vi "UHR-Fleezers Control (host) - Lorentz v2.vi"() -> ()   [LabVIEW 2014] (continued)
          shift-right: [w1383] -> _
          shift-left: 0.0 -> [w1381]
          i -> [w1390]
          stop <- w1454 stop-if-true
          w1398 = 0 ("index")
          w1419 = 1 ("dimension size")
          # "Keep phase within\n2pi so errors don't \nbuild"
          # "Accumulated\nphase"
          # "Current phase"
          # "Trap 2"
          # "Trap 1"
          # "ignore if N = 0"
          # "r"
          # "r"
          # "r"
          # "r"
          # "\"omega*t\""
          # "Trap 2"
          # "Trap separation (radians)"
          # "Trap 1"
          # "Offset (starts\n at bottom of\n the circle)"
          # "omega"
          n833 = node-c288() -> (w1467:i64)  [unwired: 1 in]
          n834 = Divide(x=w1467, y=1000) -> (x/y=w1386:dbl)
          n835 = Divide(x="2D Motion Trap Separation (MHz)", y="Radius (MHz)") -> (x/y=w1441:dbl)
          n836 = Negate(x=w1386) -> (-x=w1385:dbl)
          n837 = Divide(x="Trap 2 phase shift (deg)", y=360.0) -> (x/y=w1432:dbl)
          n838 = Inverse Sine(1:w1441) -> (0:w1377:dbl)
          n839 = Multiply(x=6.283185307179586, y=w1432) -> (x*y=w1378:dbl)
          n840 = Multiply(x=6.283185307179586, y="2D Motion Frequency (Hz)") -> (x*y=w1389:dbl)
          n841 = Select(t=w1386, s="Counterclockwise/Clockwise", f=w1385) -> (s? t:f=w1388:dbl)
          n842 = Multiply(x=w1389, y=w1388) -> (x*y=w1379:dbl)
          n843 = Select(t=w1377, s="Trap shift\nmethod", f=w1378) -> (s? t:f=w1376:dbl)
          n844 = Add(x=w1379, y=w1381) -> (x+y=w1382:dbl)
          n845 = Add(x=w1382, y=w1376) -> (x+y=w1438:dbl)
          n846 = Add(x=w1382, y=1.5707963267948966) -> (x+y=w1387:dbl)
          n847 = Add(x=w1438, y=1.5707963267948966) -> (x+y=w1451:dbl)
          n848 = Cosine(x=w1387) -> (cos(x)=w1465:dbl)
          n849 = Sine(x=w1387) -> (sin(x)=w1464:dbl)
          n850 = Multiply(x=w1465, y="Radius (MHz)") -> (x*y=w1458:dbl)
          n851 = Cosine(x=w1451) -> (cos(x)=w1463:dbl)
          n852 = Sine(x=w1451) -> (sin(x)=w1462:dbl)
          n853 = Multiply(x=w1464, y="Radius (MHz)") -> (x*y=w1457:dbl)
          n854 = Multiply(x=w1463, y="Radius (MHz)") -> (x*y=w1461:dbl)
          n855 = Multiply(x=w1462, y="Radius (MHz)") -> (x*y=w1459:dbl)
          n856 = Add(x=w1458, y=w1456) -> (x+y=w1407:dbl)
          n857 = Add(x=w1457, y=w1449) -> (x+y=w1405:dbl)
          n858 = Greater Or Equal?(x=w1390, y="N steps then stop") -> (x >= y?=w1448:bool)
          n859 = Add(x=w1461, y=w1460) -> (x+y=w1396:dbl)
          n860 = Add(x=w1459, y=w1449) -> (x+y=w1394:dbl)
          n861 = Not Equal To 0?(x="N steps then stop") -> (x != 0?=w1444:bool)
          n862 = And(x=w1448, y=w1444) -> (x .and. y?=w1445:bool)
          n863 = local read "Trap 1 sum mean"() -> (w1428:dbl)
          n864 = local read "Stop All"() -> (w1453:bool)
          n865 = local write "BD 1 Frequency 1 (MHz)"(w1407) -> ()
          n866 = local write "BD 2 Frequency 1 (MHz)"(w1405) -> ()
          n867 = local write "BD 1 Frequency 2 (MHz)"(w1396) -> ()
          n868 = local write "BD 2 Frequency 2 (MHz)"(w1394) -> ()
          n869 = Select(t=w1390, s="test", f=w1428) -> (s? t:f=→"Waveform Chart":dbl)
          n870 = Compound Arithmetic op=OR(w1453, "Stop Moving", w1445) -> (w1454:bool)
          n871 = local read "BD 1 Frequency 3 (MHz)"() -> (w1437:dbl)
          n872 = local read "BD 2 Frequency 3 (MHz)"() -> (w1436:dbl)
          n873 = Select(t=w1412, s="Reset graph", f=w1413) -> (s? t:f=w1393:dbl[])
          n874 = Select(t=w1412, s="Reset graph", f=w1414) -> (s? t:f=w1395:dbl[])
          n875 = Select(t=w1412, s="Reset graph", f=w1416) -> (s? t:f=w1404:dbl[])
          n876 = Select(t=w1412, s="Reset graph", f=w1417) -> (s? t:f=w1406:dbl[])
          n877 = Initialize Array(w1394, w1419) -> (w1420:dbl[])
          n878 = Initialize Array(w1405, w1419) -> (w1423:dbl[])
          n879 = Initialize Array(w1396, w1419) -> (w1421:dbl[])
          n880 = Initialize Array(w1407, w1419) -> (w1424:dbl[])
          n881 = local read "Y RF Frequency Limits (MHz)"() -> (w1434:T20)
          n882 = local read "X RF Frequency Limits (MHz)"() -> (w1435:T20)
          n883 = call "set RF board frequency - interlace.vi"("Board 2 Frequency Limits"=w1434, "Board 1 Frequency Limits"=w1435, "FPGA VI Reference In"=w1431, "Board 2 Frequency 3 (MHz)"=w1436, "Board 1 Frequency 3 (MHz)"=w1437, "Board 2 Frequency 2 (MHz)"=w1394, "Board 2 Frequency 1 (MHz)"=w1405, "Board 1 Frequency 2 (MHz)"=w1396, "Board 1 Frequency 1  (MHz)"=w1407) -> ()  [unwired: 1 in, 2 out]
          n884 = Bundle(w1421, w1420) -> (w1392:cluster{dbl[], dbl[]})  [unwired: 1 in]
          n885 = Bundle(w1424, w1423) -> (w1422:cluster{dbl[], dbl[]})  [unwired: 1 in]
          n886 = Build Array (concatenate)(w1407, w1406) -> (w1411:dbl[])
          n887 = Build Array (concatenate)(w1405, w1404) -> (w1409:dbl[])
          n888 = Build Array (concatenate)(w1396, w1395) -> (w1402:dbl[])
          n889 = Build Array (concatenate)(w1394, w1393) -> (w1400:dbl[])
          n890 = Bundle(w1411, w1409) -> (w1391:cluster{dbl[], dbl[]})  [unwired: 1 in]
          n891 = Bundle(w1402, w1400) -> (w1418:cluster{dbl[], dbl[]})  [unwired: 1 in]
          n892 = Build Array(w1422, w1392, w1391, w1418) -> (→"Trap trajectories":cluster{dbl[], dbl[]}[])
          n893 = case "To pause the process" shown="True" "Pause rotation" {
            frame False {
            }
            frame True {
              n894 = while {
                stop <- w1470 stop-if-true
                n895 = local read "Pause rotation"() -> (w1471:bool)
                n896 = Wait (ms)(milliseconds to wait=u32 10) -> ()  [unwired: 1 out]
                n897 = Not(x=w1471) -> (.not. x?=w1470:bool)
              }
            }
          }
          n898 = Decrement(x="N steps to plot") -> (x-1=w1397:i32)
          n899 = Array Subset(array=w1409, index=w1398, length=w1397) -> (w1408:dbl[])
          n900 = Array Subset(array=w1411, index=w1398, length=w1397) -> (w1410:dbl[])
          n901 = Array Subset(array=w1402, index=w1398, length=w1397) -> (w1401:dbl[])
          n902 = Array Subset(array=w1400, index=w1398, length=w1397) -> (w1399:dbl[])
          n903 = Quotient & Remainder(x=w1382, y=6.283185307179586) -> (x-y*floor(x/y)=w1383:dbl)  [unwired: 1 out]
          n904 = node-c288() -> ()  [unwired: 1 in, 1 out]
        }
        n905 = node-c288(w1363) -> ()  [unwired: 1 out]
        n906 = case shown="True" w1354 {
          tunnel: w1358 -> [_ w1369]
          tunnel: w1357 -> [_ w1368]
          tunnel: w1356 -> [_ w1367]
          tunnel: w1355 -> [_ w1366]
          frame False {
          }
          frame True {
            n907 = flat-sequence {
              tunnel: w1369 -> [w1373]
              tunnel: w1368 -> [w1372]
              tunnel: w1367 -> [w1371]
              tunnel: w1366 -> [w1370]
              frame #0 {
                n908 = local write "BD 1 Frequency 1 (MHz)"(w1373) -> ()
                n909 = local write "BD 2 Frequency 1 (MHz)"(w1372) -> ()
                n910 = local write "BD 1 Frequency 2 (MHz)"(w1371) -> ()
                n911 = local write "BD 2 Frequency 2 (MHz)"(w1370) -> ()
              }
              frame #1 {
                n912 = property on="Update all trap values" class="Bool (strict)"("Val(Sgnl)"=TRUE ("Value (Signaling)")) -> ()  [unwired: 2 in, 2 out]
              }
            }
          }
        }
      }
      event "Stop All": Value Change {
        # "Stopping blue laser before shutting off program"
        n913 = event-data() -> ()  [unwired: 1 in, 5 out]
        n914 = local read "Delay (ms)"() -> (w1481:i32)
        n915 = call "serial write macro.vi"("String"="l0", "Delay (ms)"=w1481, "VISA resource name"=w1484) -> ("read buffer"=w1479:string, "error out"=w1480:errorcluster, "VISA resource name out"=w1483:refnum<visa-resource-name>)
        n916 = local write "read blue buffer"(w1479) -> ()
        n917 = local write "Blue Error Out"(w1480) -> ()
        n918 = VISA Close(VISA resource name=w1483) -> ()  [unwired: 1 in, 1 out]
        n919 = local read "Stop All"() -> (w1485:bool)
      }
      event "Sensitivity", "Offset Current Sign", "Offset Current Value", "Offset Current", "Bias Voltage", "Bias Voltage (mV)", "Filter Type", "Lowpass 3dB Point", "Highpass 3dB Point", "Filter Reset", "Invert Signal", "Gain Mode", "Send Command": Value Change {
        w1492 = 250 ("Delay (ms)")
        n920 = event-data() -> ()  [unwired: 1 in, 5 out]
        n921 = event shown="[0] \"Sensitivity\": Value Change" {
          selector: _ -> [_ _ _ _ _ _ _ _ _ _ _ _ _]
          dyn-events: _ -> [_ _ _ _ _ _ _ _ _ _ _ _ _]
          timeout: _ -> [_ _ _ _ _ _ _ _ _ _ _ _ _]
          tunnel: [w1504 w1512 w1520 w1529 w1539 w1547 w1550 w1554 w1557 w1560 w1563 w1570 "Command"] -> w1491
          tunnel: [w1499 w1506 w1516 w1523 w1533 w1543 _ _ _ _ _ w1566 _] -> w1486
          event "Sensitivity": Value Change {
            n922 = event-data() -> ()  [unwired: 1 in, 5 out]
            n923 = property on="Sensitivity" class="CmbBox"() -> ("Value"=→"Gain":string)  [unwired: 2 in, 2 out]
            n924 = Concatenate Strings("SENS ", "Sensitivity") -> (w1504:string)
            n925 = local read "Gain"() -> (w1501:string)
            n926 = Concatenate Strings("gain set at ", w1501) -> (w1499:string)
          }
          event "Offset Current Sign": Value Change {
            n927 = event-data() -> ()  [unwired: 1 in, 4 out]
            n928 = Boolean To (0,1)(Boolean="Offset Current Sign") -> (0, 1=w1515:i16)
            n929 = Select(t="positive", s="Offset Current Sign", f="negative") -> (s? t:f=w1507:string)
            n930 = Number To Decimal String(number=w1515) -> (decimal integer string=w1514:string)  [unwired: 1 in]
            n931 = Concatenate Strings("IOSN " ("string"), w1514) -> (w1512:string)
            n932 = Concatenate Strings("offset current sign ", w1507) -> (w1506:string)
          }
          event "Offset Current Value": Value Change {
            n933 = event-data() -> ()  [unwired: 1 in, 5 out]
            n934 = property on="Offset Current Value" class="CmbBox"() -> ("Value"=→"Read offset current":string)  [unwired: 2 in, 2 out]
            n935 = local read "Read offset current"() -> (w1517:string)
            n936 = Concatenate Strings("IOLV ", "Offset Current Value") -> (w1520:string)
            n937 = Concatenate Strings("offset current value ", w1517) -> (w1516:string)
          }
          event "Offset Current": Value Change {
            n938 = event-data() -> ()  [unwired: 1 in, 5 out]
            n939 = Boolean To (0,1)(Boolean="Offset Current") -> (0, 1=w1532:i16)
            n940 = Select(t="on", s="Offset Current", f="off") -> (s? t:f=w1524:string)
            n941 = Number To Decimal String(number=w1532) -> (decimal integer string=w1531:string)  [unwired: 1 in]
            n942 = Concatenate Strings("IOON " ("string"), w1531) -> (w1529:string)
            n943 = Concatenate Strings("offset current ", w1524) -> (w1523:string)
          }
          event "Bias Voltage": Value Change {
            n944 = event-data() -> ()  [unwired: 1 in, 5 out]
            n945 = Boolean To (0,1)(Boolean="Bias Voltage") -> (0, 1=w1540:i16)
            n946 = Number To Decimal String(number=w1540) -> (decimal integer string=w1541:string)  [unwired: 1 in]
            n947 = Select(t="on", s="Bias Voltage", f="off") -> (s? t:f=w1534:string)
            n948 = Concatenate Strings("BSON " ("string"), w1541) -> (w1539:string)
            n949 = Concatenate Strings("bias voltage", w1534) -> (w1533:string)
          }
          event "Bias Voltage (mV)": Value Change {
            n950 = event-data() -> ()  [unwired: 1 in, 5 out]
            n951 = Number To Decimal String(number="Bias Voltage (mV)") -> (decimal integer string=w1549:string)  [unwired: 1 in]
            n952 = Number To Fractional String(number="Bias Voltage (mV)") -> (F-format string=w1544:string)  [unwired: 3 in]
            n953 = Concatenate Strings("BSLV " ("string"), w1549) -> (w1547:string)
            n954 = Concatenate Strings("bias voltage value ", w1544) -> (w1543:string)
          }
          event "Filter Type": Value Change {
            n955 = event-data() -> ()  [unwired: 1 in, 5 out]
            n956 = Concatenate Strings("FLTT " ("string"), "Filter Type") -> (w1550:string)
          }
          event "Lowpass 3dB Point": Value Change {
            n957 = event-data() -> ()  [unwired: 1 in, 5 out]
            n958 = Concatenate Strings("LFRQ " ("string"), "Lowpass 3dB Point") -> (w1554:string)
          }
          event "Highpass 3dB Point": Value Change {
            n959 = event-data() -> ()  [unwired: 1 in, 5 out]
            n960 = Concatenate Strings("HFRQ " ("string"), "Highpass 3dB Point") -> (w1557:string)
          }
          event "Filter Reset": Value Change {
            n961 = event-data() -> ()  [unwired: 1 in, 5 out]
            n962 = Select(t="ROLD", s="Filter Reset", f="") -> (s? t:f=w1560:string)
          }
          event "Gain Mode": Value Change {
            n963 = event-data() -> ()  [unwired: 1 in, 5 out]
            n964 = Concatenate Strings("GNMD " ("string"), "Gain Mode") -> (w1563:string)
          }
          event "Invert Signal": Value Change {
            n965 = event-data() -> ()  [unwired: 1 in, 5 out]
            n966 = Boolean To (0,1)(Boolean="Invert Signal") -> (0, 1=w1573:i16)
            n967 = Number To Decimal String(number=w1573) -> (decimal integer string=w1572:string)  [unwired: 1 in]
            n968 = Concatenate Strings("INVT " ("string"), w1572) -> (w1570:string)
            n969 = Select(t="signal inverted", s="Invert Signal", f="signal not inverted") -> (s? t:f=w1566:string)
          }
          event "Send Command": Value Change {
            n970 = event-data() -> ()  [unwired: 1 in, 5 out]
          }
        }
        "Command Sent" <- w1491
        n971 = local read "Save Event Log?"() -> (w1487:bool)
        n972 = local read "Saving..."() -> (w1488:bool)
        n973 = And(x=w1487, y=w1488) -> (x .and. y?=w1489:bool)
        n974 = case shown="True" w1489 {
          tunnel: w1486 -> [_ w1496]
          frame False {
          }
          frame True {
            n975 = local read "Time (s)"() -> (w1497:dbl)
            n976 = local read "log file ref"() -> (w1498:refnum<file>)
            n977 = call "write to event log.vi"("log file ref"=w1498, "time"=w1497, "input string"=w1496) -> ()  [unwired: 8 in]
          }
        }
        n978 = call "preamp serial write macro.vi"("String"=w1491, "Delay (ms)"=w1492, "VISA resource name"=w1495) -> ("read buffer"=→"Reply":string, "error out"=w1494:errorcluster)  [unwired: 1 out]
        n979 = call "preamp serial write macro.vi"("String"=w1491, "Delay (ms)"=w1492, "VISA resource name"=w1490) -> ()  [unwired: 3 out]
        n980 = local write "Preamp Error Out"(w1494) -> ()
      }
    }
    n981 = node-c288() -> ()  [unwired: 1 in, 1 out]
  }
  n982 = node-c288() -> (w30:T35)  [unwired: 4 out]
  n983 = disable-structure shown="Disabled" {
    frame Disabled {
      n984 = while "Duncan's play event loop" {
        stop <- w1577 stop-if-true
        n985 = Create User Event(user event datatype=TRUE ("Boolean")) -> (user event=w1578:refnum<user-event>)  [unwired: 1 in, 1 out]
        n986 = Create User Event(user event datatype=TRUE ("Boolean")) -> (user event=w1584:refnum<user-event>)  [unwired: 1 in, 1 out]
        n987 = global write "Global for fluorescence simulation mean (30 samples), (power series).vi" "Red Signal"(w1578) -> ()
        n988 = global write "Global for fluorescence simulation mean (30 samples), (power series).vi" "Green Signal"(w1584) -> ()
        n989 = register-events(w1584, w1578) -> (reference out=w1583:refnum<event-registration>)  [unwired: 2 in, 1 out]
        n990 = event shown="[1] \"Start assembly line\": Value Change" {
          selector: w1583 -> [_ _ _ _]
          dyn-events: _ -> [_ _ _ _]
          timeout: 100 -> [_ _ _ _]
          event Timeout {
            n991 = event-data() -> ()  [unwired: 1 in, 2 out]
          }
          event "Start assembly line": Value Change {
            n992 = event-data() -> ("OldVal"=w1586:bool)  [unwired: 1 in, 4 out]
            n993 = case shown="True" w1586 {
              selector: w1586 -> [_ w1587]
              frame False {
              }
              frame True {
                n994 = property on="Move to Position 3" class="Bool"("Val(Sgnl)"=w1587) -> ()  [unwired: 2 in, 2 out]
                n995 = case shown="1" "Numeric" {
                  frame 0, Default {
                  }
                  frame 1 {
                    n996 = property on="Green Laser ON" class="Bool (strict)"("Val(Sgnl)"=TRUE ("Value (Signaling)")) -> ()  [unwired: 2 in, 2 out]
                  }
                  frame 2 {
                    n997 = property on="Red Laser ON" class="Bool (strict)"("Val(Sgnl)"=TRUE) -> ()  [unwired: 2 in, 2 out]
                  }
                }
              }
            }
          }
          event User Event {
            n998 = event-data() -> ("Boolean"=w1591:bool)  [unwired: 1 in, 3 out]
            "Green Fluorophore" <- w1591
            n999 = property on="Start assembly line" class="Bool"("Val(Sgnl)"=w1591) -> ()  [unwired: 2 in, 2 out]
          }
          event User Event {
            n1000 = event-data() -> ("Boolean"=w1592:bool)  [unwired: 1 in, 3 out]
            "Red Fluorophore" <- w1592
            n1001 = property on="Start assembly line" class="Bool"("Val(Sgnl)"=w1592) -> ()  [unwired: 2 in, 2 out]
          }
        }
        n1002 = property on="Get Fluorophore" class="Bool (strict)"("Val(Sgnl)"="Get Fluorophore") -> ()  [unwired: 2 in, 2 out]
        n1003 = Wait (ms)(milliseconds to wait=u32 100) -> ()  [unwired: 1 out]
        n1004 = local read "Stop All"() -> (w1576:bool)
        n1005 = Or(x=w1576, y="stop") -> (x .or. y?=w1577:bool)
      }
    }
    frame Enabled {
    }
  }
  n1006 = timed-loop "Rough control of MCL mirror stage (debugging)" {
    tunnel: [w1595] -> w71
    timing: w30 -> [_]
    timing-out: [_] -> w29
    tunnel: w21 -> [w1593]
    stop <- w1595 stop-if-true
    n1007 = node-c288() -> ()  [unwired: 2 out]
    n1008 = case shown="1" "MCL Mode" {
      tunnel: w1593 -> [_ w1598 w1645]
      frame 0, Default {
      }
      frame 1 {
        n1009 = node-c288() -> (w1600:T35)  [unwired: 4 out]
        n1010 = timed-loop "Oscillate MCL mirror" {
          timing: w1600 -> [_]
          timing-out: [_] -> w1599
          tunnel: w1598 -> [w1601]
          i -> [w1639]
          stop <- w1602 stop-if-true
          n1011 = node-c288() -> (w1638:i64)  [unwired: 1 out]
          n1012 = Multiply(x="AO1", y=32767.0) -> (x*y=w1634:dbl)
          n1013 = Multiply(x="AO2", y=32767.0) -> (x*y=w1629:dbl)
          n1014 = Divide(x=w1634, y=10.0) -> (x/y=w1635:dbl)
          n1015 = Divide(x=w1629, y=10.0) -> (x/y=w1630:dbl)
          n1016 = To Word Integer(number=w1635) -> (16bit integer=w1627:i16)
          n1017 = To Word Integer(number=w1630) -> (16bit integer=w1626:i16)
          n1018 = Divide(x=w1638, y=i64 1000) -> (x/y=w1609:dbl)
          n1019 = Multiply(x=w1609, y=w1639) -> (x*y=w1620:dbl)
          n1020 = Multiply(x="Osc. freq. (Hz) 2", y=6.283185307179586) -> (x*y=w1621:dbl)
          n1021 = Multiply(x=w1621, y=w1620) -> (x*y=w1619:dbl)
          n1022 = Sine(x=w1619) -> (sin(x)=w1618:dbl)
          n1023 = Multiply(x=w1618, y="Osc. amp. (V)") -> (x*y=w1616:dbl)
          n1024 = Add(x=w1616, y="Osc. center (V)") -> (x+y=w1614:dbl)
          n1025 = Divide(x=w1614, y=10.0) -> (x/y=w1612:dbl)
          n1026 = Multiply(x=w1612, y=32767.0) -> (x*y=w1607:dbl)
          n1027 = Select(t=w1607, s="Scan axis", f=w1627) -> (s? t:f=w1625:dbl)
          n1028 = Select(t=w1626, s="Scan axis", f=w1607) -> (s? t:f=w1624:dbl)
          n1029 = local read "MCL Mode"() -> (w1606:u16)
          n1030 = Not Equal?(x=w1606, y=u16 1) -> (x != y?=w1603:bool)
          n1031 = local read "Stop All"() -> (w1604:bool)
          n1032 = xnode "Read/Write Control"("FPGA VI Reference In"=w1601, "AO1"=w1625, "AO2"=w1624) -> ()  [unwired: 1 in, 2 out]
          n1033 = Compound Arithmetic op=OR(w1604, w1603) -> (w1602:bool)
          n1034 = node-c288() -> ()  [unwired: 2 out]
        }
        n1035 = node-c288(w1599) -> ()  [unwired: 1 out]
      }
      frame 2 {
        n1036 = case shown="True" "Start Scan" {
          tunnel: w1645 -> [_ w1647]
          frame False {
          }
          frame True {
            n1037 = Subtract(x="End (V)", y="Begin (V)") -> (x-y=w1654:dbl)
            n1038 = Decrement(x="N Points") -> (x-1=w1653:dbl)
            n1039 = Divide(x=w1654, y=w1653) -> (x/y=w1651:dbl)
            n1040 = for {
              N: "N Points" -> [_]
              tunnel: "Begin (V)" -> [w1670]
              tunnel: [w1662] -> w1657 mode=indexing
              tunnel: w1651 -> [w1661]
              tunnel: [w1659] -> w1650 mode=indexing
              tunnel: w1647 -> [w1658]
              i -> [w1669]
              n1041 = Multiply(x=w1661, y=w1669) -> (x*y=w1668:dbl)
              n1042 = Add(x=w1670, y=w1668) -> (x+y=w1665:dbl)
              n1043 = local read "Scan axis"() -> (w1660:bool)
              n1044 = local read "AO1"() -> (w1667:dbl)
              n1045 = local read "AO2"() -> (w1666:dbl)
              n1046 = Select(t=w1665, s=w1660, f=w1667) -> (s? t:f=w1664:dbl)
              n1047 = Select(t=w1666, s=w1660, f=w1665) -> (s? t:f=w1663:dbl)
              n1048 = flat-sequence {
                tunnel: w1664 -> [w1674]
                tunnel: w1663 -> [w1673]
                tunnel: w1658 -> [w1671]
                tunnel: [w1684] -> w1662
                tunnel: [w1683] -> w1659
                frame #0 {
                  w1677 = 10.0 ("y")
                  w1672 = 32767.0 ("y")
                  n1049 = Multiply(x=w1674, y=w1672) -> (x*y=w1680:dbl)
                  n1050 = Multiply(x=w1673, y=w1672) -> (x*y=w1678:dbl)
                  n1051 = Divide(x=w1680, y=w1677) -> (x/y=w1681:dbl)
                  n1052 = Divide(x=w1678, y=w1677) -> (x/y=w1679:dbl)
                  n1053 = To Word Integer(number=w1681) -> (16bit integer=w1675:i16)
                  n1054 = To Word Integer(number=w1679) -> (16bit integer=w1676:i16)
                  n1055 = xnode "Read/Write Control"("FPGA VI Reference In"=w1671, "AO1"=w1675, "AO2"=w1676) -> ()  [unwired: 1 in, 2 out]
                }
                frame #1 {
                  n1056 = Wait (ms)(milliseconds to wait="DAQ Delay (ms)") -> ()  [unwired: 1 out]
                }
                frame #2 {
                  n1057 = local read "Slow mean"() -> (w1684:dbl)
                  n1058 = local read "Sigma"() -> (w1683:dbl)
                }
              }
            }
            n1059 = Bundle("Begin (V)"="Begin (V)", w1651, w1657) -> (→"MCL Scan":cluster{"Begin (V)":dbl, dbl, dbl[]})  [unwired: 1 out]
            n1060 = Bundle("Begin (V)"="Begin (V)", w1651, w1650) -> (→"MCL Scan 2":cluster{"Begin (V)":dbl, dbl, dbl[]})  [unwired: 1 out]
          }
        }
      }
    }
    n1061 = local read "Stop All"() -> (w1595:bool)
    n1062 = node-c288() -> ()  [unwired: 2 out]
  }
  n1063 = node-c288(2 ("Processor")) -> (w62:T35)  [unwired: 3 out]
  n1064 = timed-loop "Basic control parameters (all FPGA settings, other basic controls)" {
    shift-right: [w1692] -> _
    shift-left: errorcluster {"status"=FALSE, "code"=0, "source"=""} ("error out") -> [_]
    tunnel: [w1691] -> _
    timing: w62 -> [_]
    timing-out: [_] -> w61
    tunnel: w43 -> [w1690]
    tunnel: w39 -> [w1689]
    tunnel: w38 -> [w1688]
    tunnel: w37 -> [w1687]
    tunnel: w36 -> [w1686]
    tunnel: w21 -> [w1685]
    stop <- w1691 stop-if-true
    n1065 = node-c288() -> ()  [unwired: 2 out]
    n1066 = event shown="[71] \"Trap Pos. FB Range\", \"Trap Pos. FB Gains\", \"Trap Pos. FB Mult Factor\", \"Trap Pos. FB Offset Factor\", \"Trap Pos FB Negate Action\", \"Trap Pos FB Monitor T1 or T2\", \"Differential FB?\", \"Negate Diff?\": Value Change" {
      selector: _ -> [_ _ _ _ _ _ _ _ _ _ _ _ _ _ _ _ _ _ _ _ _ _ _ _ _ _ _ _ _ _ _ _ _ _ _ _ _ _ _ _ _ _ _ _ _ _ _ _ _ _ _ _ _ _ _ _ _ _ _ _ _ _ _ _ _ _ _ _ _ _ _ _ _ _ _ _ _ _ _ _ _ _ _ _ _ _ _]
      dyn-events: _ -> [_ _ _ _ _ _ _ _ _ _ _ _ _ _ _ _ _ _ _ _ _ _ _ _ _ _ _ _ _ _ _ _ _ _ _ _ _ _ _ _ _ _ _ _ _ _ _ _ _ _ _ _ _ _ _ _ _ _ _ _ _ _ _ _ _ _ _ _ _ _ _ _ _ _ _ _ _ _ _ _ _ _ _ _ _ _ _]
      timeout: _ -> [_ _ _ _ _ _ _ _ _ _ _ _ _ _ _ _ _ _ _ _ _ _ _ _ _ _ _ _ _ _ _ _ _ _ _ _ _ _ _ _ _ _ _ _ _ _ _ _ _ _ _ _ _ _ _ _ _ _ _ _ _ _ _ _ _ _ _ _ _ _ _ _ _ _ _ _ _ _ _ _ _ _ _ _ _ _ _]
      tunnel: [w1732 _ _ _ w1762 _ _ _ _ _ _ _ w1868 _ _ w1955 w1957 w1964 w1966 w2036 _ w2078 w2104 w2132 w2157 w2184 w2210 w2239 _ w2244 w2338 w2342 w2379 _ w2442 w2445 w2448 w2458 w2461 _ w2468 _ _ _ _ _ _ _ _ _ _ _ _ _ _ _ _ _ _ _ _ w2965 _ _ _ _ w3001 _ _ _ _ _ _ _ _ _ _ _ _ _ _ _ _ _ _ w3282 _] -> w1692
      tunnel: [_ _ _ _ _ _ _ _ _ _ w1847 _ _ _ _ _ _ _ _ _ _ _ _ _ _ _ _ _ _ _ _ _ _ _ _ _ _ _ _ _ _ _ _ _ _ _ _ _ _ _ _ _ _ _ _ _ _ _ _ _ _ _ _ _ _ _ _ _ _ _ _ _ _ _ _ _ _ _ _ _ _ _ _ _ _ _ _] -> w1691
      tunnel: [_ _ _ _ _ _ _ _ "Round T1 X" _ _ _ _ _ _ _ _ _ _ _ _ _ _ _ _ _ _ _ _ _ _ _ _ _ _ _ _ _ _ _ _ _ _ _ _ _ _ _ _ _ _ _ _ _ _ _ _ _ _ _ _ _ _ _ _ _ _ _ _ _ _ _ _ _ _ _ _ _ _ _ _ _ _ _ _ _ _] -> _
      tunnel: [_ _ _ "Adjust Scale\nto Mean" _ _ _ _ _ _ _ _ _ _ _ _ _ _ _ _ _ _ _ _ _ _ _ _ _ "Test ttrig" _ _ _ _ _ _ _ _ _ _ _ _ _ _ _ _ _ _ _ _ _ w2712 w2776 w2823 w2872 _ _ _ _ _ _ _ _ _ _ _ _ _ _ _ _ _ _ _ _ _ _ _ _ _ _ _ _ _ _ _ _] -> _
      tunnel: [_ _ _ _ _ _ _ _ _ "Round T2 X" _ "Delayed Interlace Start" _ _ _ _ _ _ _ _ _ _ _ _ _ _ _ _ _ _ _ _ _ _ _ _ _ _ _ _ _ _ _ _ _ _ _ _ _ _ _ _ _ _ _ _ _ _ _ _ _ _ _ _ _ _ _ _ _ _ _ _ _ _ _ _ _ _ _ _ _ _ _ _ _ _ _] -> _
      tunnel: w1690 -> [_ _ _ _ _ _ _ _ _ _ _ _ _ _ _ _ _ _ _ _ _ _ _ _ _ _ _ _ _ _ _ _ _ _ _ _ _ _ _ _ _ _ _ _ _ _ _ w2682 w2690 w2697 w2703 w2711 _ _ w2871 _ _ _ _ _ _ _ _ _ _ _ _ _ _ _ _ _ _ _ _ _ _ _ _ _ _ _ _ _ _ _ _]
      tunnel: w1689 -> [_ _ _ _ _ _ _ _ _ _ _ _ _ _ _ _ _ _ _ _ _ _ _ _ _ _ _ _ _ _ _ _ _ _ _ _ _ _ _ _ _ _ _ _ _ w2569 _ _ _ _ _ _ w2775 _ _ w2878 _ w2890 _ w2906 _ _ _ _ _ _ _ _ _ _ _ _ _ _ _ _ _ _ _ _ _ _ _ _ _ _ _]
      tunnel: w1688 -> [_ _ _ _ _ _ _ _ _ _ _ _ _ _ _ _ _ _ _ _ _ _ _ _ _ _ _ _ _ _ _ _ _ _ _ _ _ _ _ _ _ _ _ _ _ _ _ _ _ _ _ _ _ _ _ _ _ _ _ _ _ _ _ _ _ _ _ _ _ _ _ _ _ _ _ _ _ _ _ _ _ _ _ _ _ _ _]
      tunnel: w1687 -> [_ _ _ _ _ _ _ _ _ _ _ _ _ _ _ _ _ _ _ _ _ _ _ _ _ _ _ _ _ _ _ _ _ _ _ _ _ _ _ _ _ w2479 _ _ _ _ _ _ _ _ _ _ _ w2822 _ _ w2884 _ w2898 _ w2932 _ _ _ _ _ _ _ _ _ _ _ _ _ _ _ _ _ _ _ _ _ _ _ _ _ _]
      tunnel: w1686 -> [_ _ _ _ _ _ _ _ _ _ _ _ _ _ _ _ _ _ _ _ _ _ _ _ _ _ _ _ _ _ _ _ _ _ _ _ _ _ _ _ _ _ _ _ _ _ _ _ _ _ _ _ _ _ _ _ _ _ _ _ _ _ _ _ _ _ _ _ _ _ _ _ _ _ _ _ _ _ _ _ _ _ _ _ _ _ _]
      tunnel: w1685 -> [w1695 _ _ _ w1761 _ w1787 _ _ _ _ _ w1859 _ _ w1937 w1956 w1963 w1965 w2001 _ w2067 w2102 w2114 w2139 w2167 w2187 w2215 w2240 w2242 w2246 w2339 w2343 _ w2439 w2443 w2446 w2456 w2459 _ w2467 _ _ _ _ _ _ _ _ _ _ _ _ _ _ _ _ _ _ _ _ w2958 _ w2979 _ w2985 w3000 _ w3007 w3034 w3041 w3057 w3065 _ w3076 _ w3120 _ _ w3174 w3205 w3209 w3217 _ w3281 _ w3288]
      tunnel: [_ _ _ _ _ _ _ _ _ _ w1846 _ _ _ _ _ _ _ _ _ _ _ _ _ _ _ _ _ _ _ _ _ _ _ _ _ _ _ _ _ _ _ w2557 w2561 w2565 _ _ _ _ _ _ _ _ _ _ _ _ _ _ _ _ _ _ _ _ _ _ _ _ _ _ _ _ _ _ _ _ _ _ _ _ _ _ _ _ _ _] -> _
      event "AI Count (ticks)", "Sets to FIFO (Traps)", "Save ave N", "FPGA Ave.", "# Samples/channel", "N sets to save": Value Change {
        # "So that if 'Save ave N' is updated, the AOD scanning code updates too."
        n1067 = event-data() -> ()  [unwired: 6 out]
        n1068 = local read "AI Count (ticks)"() -> (w1716:u16)
        n1069 = Unbundle By Name("Sets to FIFO (Traps)") -> ("Set 1"=w1699:bool, "Set 2"=w1698:bool, "Set 3"=w1697:bool)
        n1070 = Boolean To (0,1)(Boolean="Sets to FIFO (Traps)") -> (0, 1=w1724:cluster{"Set 1":i16, "Set 2":i16, "Set 3":i16})
        n1071 = xnode "Read/Write Control"("FPGA VI Reference In"=w1695, "ai count"=w1716, "Set 1"=w1699, "Set 2"=w1698, "Set 3"=w1697, "N of AI1 Int Acq Sets"="N Acq Sets (Traps + Fl.)") -> ("error out"=w1732:errorcluster)  [unwired: 1 in, 1 out]
        n1072 = Cluster To Array(cluster=w1724) -> (array=w1723:i16[])
        n1073 = To Unsigned Long Integer(number=w1723) -> (unsigned 32bit integer=w1705:u32[])
        n1074 = local read "Scan steps (AOD)"() -> (w1725:u64)
        n1075 = Multiply(x=w1716, y="N Acq Sets (Traps + Fl.)") -> (x*y=w1714:u16)
        n1076 = Divide(x=40000000.0, y=w1716) -> (x/y=w1708:dbl)
        "AI rate (Hz)" <- w1708
        "Ave. Rate (Hz)" <- w1708
        n1077 = Add Array Elements(numeric array=w1705) -> (sum=w1717:u32)
        "Trap Sets" <- w1717
        n1078 = Reciprocal(x=w1708) -> (1/x=→"Ave. Period (s)":dbl)
        n1079 = property on="Scan steps (AOD)" class="DigNum (strict)"("Val(Sgnl)"=w1725) -> ()  [unwired: 2 in, 2 out]
        n1080 = Divide(x=w1708, y="N Acq Sets (Traps + Fl.)") -> (x/y=w1729:dbl)
        "Data Rate (Hz)" <- w1729
        n1081 = Reciprocal(x=w1729) -> (1/x=→"Data Period (s)":dbl)
        n1082 = local read "Save ave N"() -> (w1728:dbl)
        n1083 = Divide(x=w1729, y=w1728) -> (x/y=w1727:dbl)
        "Save Data Rate (Hz)" <- w1727
        n1084 = Reciprocal(x=w1727) -> (1/x=→"Save Data Period (s)":dbl)
        n1085 = Multiply(x=w1714, y="# Samples/trap") -> (x*y=w1712:u32)
        "Counts/DMA" <- w1712
        n1086 = property on="Trap Disp. Downsample" class="DigNum (strict)"("Maximum"="# Samples/trap") -> ()  [unwired: 2 in, 2 out]
        n1087 = Multiply(x=w1717, y="# Samples/trap") -> (x*y=w1706:u32)
        "# Samples/channel" <- w1706
        n1088 = Multiply(x=w1706, y=u32 8) -> (x*y=→"Trap AI Elements/DMA read":u32)
        n1089 = local read "APD Int. Count"() -> (w1713:u32)
        n1090 = Multiply(x=w1706, y=u32 3) -> (x*y=→"Trap Pos Elements/DMA read":u32)
        n1091 = Divide(x=w1712, y=w1713) -> (x/y=w1703:dbl)
        "APD Samples/FIFO Acq." <- w1703
        n1092 = Divide(x=w1712, y=40000000.0) -> (x/y=w1710:dbl)
        "DMA Update Period (s)" <- w1710
        n1093 = local read "Number of APDs"() -> (w1696:u8)
        n1094 = Multiply(x=w1696, y=w1703) -> (x*y=→"APD Elements/DMA read":dbl)
        n1095 = property on="APD Disp. Downsample" class="DigNum (strict)"("Maximum"=w1703) -> ()  [unwired: 2 in, 2 out]
        n1096 = local read "N sets to save"() -> (w1722:u32)
        n1097 = Multiply(x=w1710, y=w1722) -> (x*y=→"Total Time (s) 2":dbl)
        "FPGA Averaging" <- FALSE ("FPGA Averaging")
      }
      event "Remove Offset": Value Change {
        n1098 = event-data() -> ()  [unwired: 7 out]
        n1099 = local write "Remove Offset"(FALSE ("Remove Offset")) -> ()
        n1100 = local read "Bead Mean (nm)"() -> (w1734:dbl)
        n1101 = local read "Offset (nm)"() -> (w1735:dbl)
        n1102 = Add(x=w1734, y=w1735) -> (x+y=w1733:dbl)
        n1103 = local write "Offset (nm)"(w1733) -> ()
        n1104 = disable-structure shown="Disabled" {
          frame Disabled {
            n1105 = local read "Bead Mean (nm)"() -> (w1740:dbl)
            n1106 = Add(y=w1740) -> (x=w1739:dbl, x+y=w1738:dbl)
            n1107 = Subtract(x=w1740, y=w1739) -> (x-y=w1737:dbl)
            n1108 = property on="Bead Separation" class="WFChart (strict)"("YScale.Minimum"=w1737) -> ()  [unwired: 2 in, 2 out]
            n1109 = property on="Bead Separation" class="WFChart (strict)"("YScale.Maximum"=w1738) -> ()  [unwired: 2 in, 2 out]
          }
          frame Enabled {
          }
        }
      }
      event "Detector Type": Value Change {
        n1110 = event-data() -> ()  [unwired: 7 out]
        n1111 = local read "AI labels"() -> (w1742:string[])
        n1112 = property on="High Res. Display" class="Ring (strict)"("Strings []"=w1742) -> ()  [unwired: 2 in, 2 out]
        n1113 = Build Array (concatenate)(w1742, "none") -> (w1743:string[])
        n1114 = property on="FFT 1 Choice 1" class="Ring (strict)"("Strings []"=w1743) -> ()  [unwired: 2 in, 2 out]
        n1115 = property on="FFT 1 Choice 2" class="Ring (strict)"("Strings []"=w1743) -> ()  [unwired: 2 in, 2 out]
        n1116 = property on="FFT 2 Choice 1" class="Ring (strict)"("Strings []"=w1743) -> ()  [unwired: 2 in, 2 out]
        n1117 = property on="FFT 2 Choice 2" class="Ring (strict)"("Strings []"=w1743) -> ()  [unwired: 2 in, 2 out]
        n1118 = Bundle("APD 1", "APD 2", "APD 3") -> (w1746:cluster{string, string, string})  [unwired: 1 out]
        n1119 = Cluster To Array(cluster=w1746) -> (array=w1744:string[])
        n1120 = Build Array (concatenate)(w1744, w1743) -> (w1748:string[])
        n1121 = Array Size(array=w1748) -> (size(s)=w1749:i32)
        n1122 = property on="Signals to Plot" class="LstBox (strict)"("Item Names"=w1748) -> ()  [unwired: 2 in, 2 out]
        n1123 = property on="Signals to Plot" class="LstBox (strict)"("Number of Rows"=w1749) -> ()  [unwired: 2 in, 2 out]
        n1124 = property on="All Signals" class="WFChart (strict)"("LegNumRows"=w1749) -> ()  [unwired: 2 in, 2 out]
      }
      event "Adjust Scale\nto Mean": Value Change {
        n1125 = event-data() -> ()  [unwired: 7 out]
        n1126 = local read "APD 1 Rate (Hz)"() -> (w1758:dbl)
        n1127 = Multiply(x=1000.0, y="Above (kHz)") -> (x*y=w1756:dbl)
        n1128 = Multiply(x=1000.0, y="Below (kHz)") -> (x*y=w1754:dbl)
        n1129 = Add(x=w1756, y=w1758) -> (x+y=w1751:dbl)
        n1130 = Subtract(x=w1758, y=w1754) -> (x-y=w1752:dbl)
        n1131 = property on="APD Chart" class="WFChart (strict)"("YScale.Minimum"=w1752) -> ()  [unwired: 2 in, 2 out]
        n1132 = property on="APD Chart" class="WFChart (strict)"("YScale.Maximum"=w1751) -> ()  [unwired: 2 in, 2 out]
      }
      event "Phase adj. (AI1)", "+ phase (AI1)", "- phase (AI1)": Value Change {
        n1133 = event-data() -> ()  [unwired: 7 out]
        n1134 = Negate(x="Phase adj. (AI1)") -> (-x=w1769:i16)
        n1135 = Select(t=w1769, s="- phase (AI1)", f="Phase adj. (AI1)") -> (s? t:f=w1768:i16)
        n1136 = xnode "Read/Write Control"("FPGA VI Reference In"=w1761, "Phase count adjustment"=w1768) -> ("FPGA VI Reference Out"=w1767:T31, "error out"=w1766:errorcluster)  [unwired: 2 in]
        n1137 = Or(x="- phase (AI1)", y="+ phase (AI1)") -> (x .or. y?=w1763:bool)
        n1138 = xnode "Read/Write Control"("FPGA VI Reference In"=w1767, "error in"=w1766, "+ phase"=w1763) -> ("error out"=w1762:errorcluster)  [unwired: 1 in, 1 out]
      }
      event "Signals to Plot": Double Click {
        w1773 = u32 9868950 ("Color Box")
        n1139 = event-data() -> ("Row"=w1775:i32)  [unwired: 9 out]
        n1140 = property on="All Signals" class="WFChart (strict)"("Active Plot"=w1775) -> (error out=w1786:errorcluster)  [unwired: 2 in, 1 out]
        n1141 = property on="All Signals" class="WFChart (strict)" props=["Plot", "Visible?", "Plot", "Plot Color"](error in=w1786) -> (error out=w1785:errorcluster, "Plot.Visible?"=w1784:bool)  [unwired: 1 in, 2 out]
        n1142 = Select(t=FALSE ("Plot.Visible"), s=w1784, f=TRUE ("Plot.Visible")) -> (s? t:f=w1779:bool)
        n1143 = property on="All Signals" class="WFChart (strict)"(error in=w1785, "Plot.Visible?"=w1779) -> (error out=w1781:errorcluster)  [unwired: 1 in, 1 out]
        n1144 = property on="All Signals" class="WFChart (strict)"(error in=w1781) -> (error out=w1776:errorcluster, "Plot.Plot Color"=w1780:u32)  [unwired: 1 in, 1 out]
        n1145 = property on="Signals to Plot" class="LstBox (strict)"(error in=w1776, "Active Row"=w1775) -> (error out=w1774:errorcluster)  [unwired: 1 in, 1 out]
        n1146 = Select(t=w1780, s=w1779, f=u32 0) -> (s? t:f=w1777:u32)
        n1147 = property on="Signals to Plot" class="LstBox (strict)"(error in=w1774, "CellFontColor"=w1777, "SelColor"=w1773, "CellBG"=w1773, "CellFontSize"=u32 20 ("Active Row:Cell Font:Size"), "CellFontBold"=TRUE ("Active Row:Cell Font:Bold")) -> ()  [unwired: 1 in, 2 out]
      }
      event "BD 1 Frequency 1 (MHz)", "BD 1 Frequency 2 (MHz)", "BD 1 Frequency 3 (MHz)", "BD 2 Frequency 1 (MHz)", "BD 2 Frequency 2 (MHz)", "BD 2 Frequency 3 (MHz)", "Trap Delta (MHz)", "Update all trap values": Value Change {
        # "This is so you can set trap frequencies\nvia local variables and then update\nall at once"
        n1148 = event-data() -> ("CtlRef"=w1791:refnum<vi>)  [unwired: 6 out]
        n1149 = control-ref of="Trap Delta (MHz)"() -> (w1790:refnum<vi>)
        n1150 = Equal?(x=w1790, y=w1791) -> (x = y?=w1789:bool)
        n1151 = local write "Update all trap values"(FALSE ("Update all trap values")) -> ()
        n1152 = case shown="False" "Oscillate Set 1" {
          tunnel: w1789 -> [w1805 _]
          tunnel: w1787 -> [w1803 _]
          frame False {
            n1153 = local read "BD 1 Frequency 2 (MHz)"() -> (w1801:dbl)
            n1154 = case shown="False" "Symmetric?" {
              tunnel: "Trap Delta (MHz)" -> [w1827 w1834]
              tunnel: [w1828 w1832] -> w1793
              tunnel: [w1826 w1829] -> w1795
              tunnel: w1801 -> [w1828 _]
              frame False {
                n1155 = Subtract(x=w1828, y=w1827) -> (x-y=w1826:dbl)
              }
              frame True {
                w1831 = 75
                n1156 = Divide(x=w1834, y=2.0) -> (x/y=w1830:dbl)
                n1157 = Add(x=w1830, y=w1831) -> (x+y=w1832:dbl)
                n1158 = Subtract(x=w1831, y=w1830) -> (x-y=w1829:dbl)
              }
            }
            n1159 = local read "BD 1 Frequency 1 (MHz)"() -> (w1796:dbl)
            n1160 = Not(x="Symmetric?") -> (.not. x?=w1799:bool)
            n1161 = And(x=w1799, y="move Con X?") -> (x .and. y?=w1797:bool)
            n1162 = Subtract(x=w1796, y=w1795) -> (x-y=w1794:dbl)
            n1163 = Select(t=w1795, s=w1805, f=w1796) -> (s? t:f=w1804:dbl)
            n1164 = local read "Y RF Frequency Limits (MHz)"() -> (w1806:T20)
            n1165 = case shown="True" w1797 {
              tunnel: w1794 -> [_ w1825]
              frame False {
              }
              frame True {
                n1166 = property on="AOM X Cal (nm/MHz)" class="DigNum (strict)"() -> ("Value"=w1824:dbl)  [unwired: 2 in, 2 out]
                n1167 = property on="MCL Step Position Ratio" class="DigNum (strict)"() -> ("Value"=w1818:dbl)  [unwired: 2 in, 2 out]
                n1168 = Compound Arithmetic op=MULTIPLY(w1825, w1824, w1818) -> (w1823:dbl)
                n1169 = property on="MCL X Cal (nm/V)" class="DigNum (strict)"() -> ("Value"=w1822:dbl)  [unwired: 2 in, 2 out]
                n1170 = Divide(x=w1823, y=w1822) -> (x/y=w1821:dbl)
                n1171 = property on="AO2" class="Slide (strict)"() -> ("Value"=w1820:dbl)  [unwired: 2 in, 2 out]
                n1172 = Add(x=w1821, y=w1820) -> (x+y=w1819:dbl)
                n1173 = property on="AO2" class="Slide (strict)"("Val(Sgnl)"=w1819) -> ()  [unwired: 2 in, 2 out]
              }
            }
            n1174 = local read "X RF Frequency Limits (MHz)"() -> (w1807:T20)
            n1175 = local write "BD 1 Frequency 1 (MHz)"(w1804) -> ()
            n1176 = local read "BD 1 Frequency 3 (MHz)"() -> (w1816:dbl)
            n1177 = local read "BD 2 Frequency 1 (MHz)"() -> (w1810:dbl)
            n1178 = local read "BD 2 Frequency 2 (MHz)"() -> (w1809:dbl)
            n1179 = local read "BD 2 Frequency 3 (MHz)"() -> (w1817:dbl)
            n1180 = call "set RF board frequency - interlace.vi"("Board 2 Frequency Limits"=w1806, "Board 1 Frequency Limits"=w1807, "FPGA VI Reference In"=w1803, "Board 2 Frequency 3 (MHz)"=w1817, "Board 1 Frequency 3 (MHz)"=w1816, "Board 2 Frequency 2 (MHz)"=w1809, "Board 2 Frequency 1 (MHz)"=w1810, "Board 1 Frequency 2 (MHz)"=w1793, "Board 1 Frequency 1  (MHz)"=w1804) -> ()  [unwired: 1 in, 2 out]
            n1181 = Subtract(x=w1810, y=w1809) -> (x-y=w1814:dbl)
            n1182 = local write "BD 1 Frequency 2 (MHz)"(w1793) -> ()
            n1183 = Subtract(x=w1804, y=w1793) -> (x-y=w1815:dbl)
            n1184 = Square(x=w1814) -> (x^2=w1812:dbl)
            n1185 = Square(x=w1815) -> (x^2=w1813:dbl)
            n1186 = Add(x=w1813, y=w1812) -> (x+y=w1811:dbl)
            n1187 = Square Root(x=w1811) -> (sqrt(x)=w1808:dbl)
            n1188 = property on="Initial delta (MHz)" class="DigNum (strict)"("Val(Sgnl)"=w1808) -> ()  [unwired: 2 in, 2 out]
            n1189 = local write "Trap Delta (MHz)"(w1808) -> ()
          }
          frame True {
          }
        }
      }
      event "manual raster set": Value Change {
        n1190 = event-data() -> ()  [unwired: 7 out]
        n1191 = flat-sequence {
          frame #0 {
            n1192 = Replace Array Subset(array=u32[] [0] ("Index Values"), new element="manual raster set", index=0) -> (w1835:u32[])
            n1193 = property on="Saved AOD Raster Scan Parameter Sets" class="Arr (strict)"("Index Values"=w1835) -> ()  [unwired: 2 in, 2 out]
          }
          frame #1 {
            n1194 = property on="Load parameters" class="Bool (strict)"("Val(Sgnl)"=TRUE ("Value (Signaling)")) -> ()  [unwired: 2 in, 2 out]
          }
        }
      }
      event "Round T1 X": Value Change {
        n1195 = event-data() -> ()  [unwired: 7 out]
        n1196 = local read "BD 1 Frequency 1 (MHz)"() -> (w1842:dbl)
        n1197 = Round To Nearest(number=w1842) -> (nearest integer value=w1841:dbl)
        n1198 = property on="BD 1 Frequency 1 (MHz)" class="DigNum (strict)"("Val(Sgnl)"=w1841) -> ()  [unwired: 2 in, 2 out]
      }
      event "Round T2 X": Value Change {
        n1199 = event-data() -> ()  [unwired: 7 out]
        n1200 = local read "BD 1 Frequency 2 (MHz)"() -> (w1844:dbl)
        n1201 = Round To Nearest(number=w1844) -> (nearest integer value=w1843:dbl)
        n1202 = property on="BD 1 Frequency 2 (MHz)" class="DigNum (strict)"("Val(Sgnl)"=w1843) -> ()  [unwired: 2 in, 2 out]
      }
      event "Stop All": Value Change {
        n1203 = event-data() -> ()  [unwired: 7 out]
        n1204 = flat-sequence {
          tunnel: [w1849] -> w1848
          tunnel: [w1853] -> w1846
          tunnel: w1848 -> [w1853]
          tunnel: [TRUE] -> _
          tunnel: [w1851] -> w1847
          frame #0 {
            n1205 = call "hamilton_controller.vi"("action"=T32."DISCONNECT") -> ("error out"=w1849:errorcluster)  [unwired: 9 in, 1 out]
          }
          frame #1 {
            n1206 = local read "Stop All"() -> (w1851:bool)
          }
        }
      }
      event "Delayed Interlace Start": Value Change {
        n1207 = event-data() -> ()  [unwired: 7 out]
        n1208 = flat-sequence {
          frame #0 {
            n1209 = Multiply(x="Delay to Interlace (s)", y=1000.0) -> (x*y=w1855:dbl)
            n1210 = Wait (ms)(milliseconds to wait=w1855) -> ()  [unwired: 1 out]
          }
          frame #1 {
            n1211 = property on="Laser interlacing mode" class="RadioBtnsControl (strict)"("Val(Sgnl)"=enum32{"Laser ON", "Laser OFF", "Interlace"}."Interlace" ("Value (Signaling)")) -> ()  [unwired: 2 in, 2 out]
          }
        }
      }
      event "BD 1 Amplitude 1 (%)", "BD 1 Amplitude 2 (%)", "BD 1 Amplitude 3 (%)", "BD 2 Amplitude 1 (%)", "BD 2 Amplitude 2 (%)", "BD 2 Amplitude 3 (%)", "Trap 1 ON", "Trap 2 ON", "Trap 3 ON", "Feedback On/Off", "All FB On/Off": Value Change {
        w1880 = i16 1 ("f")
        n1212 = event-data() -> ()  [unwired: 7 out]
        n1213 = local write "Trap 1 (ON/OFF)"("Trap 1 ON") -> ()
        n1214 = local write "Trap 2 (ON/OFF)"("Trap 2 ON") -> ()
        n1215 = Boolean To (0,1)(Boolean="Trap 3 ON") -> (0, 1=w1881:i16)
        n1216 = Boolean To (0,1)(Boolean="Trap 1 ON") -> (0, 1=w1882:i16)
        n1217 = Boolean To (0,1)(Boolean="Trap 2 ON") -> (0, 1=w1883:i16)
        n1218 = Select(t=w1883, s="Trap ON/OFF X or Y Amp?", f=w1880) -> (s? t:f=w1878:i16)
        n1219 = Select(t=w1882, s="Trap ON/OFF X or Y Amp?", f=w1880) -> (s? t:f=w1879:i16)
        n1220 = Select(t=w1881, s="Trap ON/OFF X or Y Amp?", f=w1880) -> (s? t:f=w1877:i16)
        n1221 = Select(t=w1880, s="Trap ON/OFF X or Y Amp?", f=w1883) -> (s? t:f=w1875:i16)
        n1222 = Select(t=w1880, s="Trap ON/OFF X or Y Amp?", f=w1882) -> (s? t:f=w1876:i16)
        n1223 = Select(t=w1880, s="Trap ON/OFF X or Y Amp?", f=w1881) -> (s? t:f=w1874:i16)
        n1224 = And(x="All FB On/Off", y="Feedback On/Off") -> (x .and. y?=w1872:cluster{"Set 1":bool, "Set 2":bool})
        n1225 = local read "BD 1 Amplitude 1 (%)"() -> (w1890:dbl)
        n1226 = local read "BD 1 Amplitude 2 (%)"() -> (w1889:dbl)
        n1227 = local read "BD 1 Amplitude 3 (%)"() -> (w1888:dbl)
        n1228 = Unbundle By Name(w1872) -> ("Set 1"=w1867:bool, "Set 2"=w1864:bool)
        n1229 = local read "Y RF Amplitude Limits (%)"() -> (w1860:T20)
        n1230 = local read "X RF Amplitude Limits (%)"() -> (w1861:T20)
        n1231 = local read "BD 2 Amplitude 1 (%)"() -> (w1891:dbl)
        n1232 = local read "BD 2 Amplitude 2 (%)"() -> (w1892:dbl)
        n1233 = local read "BD 2 Amplitude 3 (%)"() -> (w1893:dbl)
        n1234 = And(x="Trap 2 ON", y=w1864) -> (x .and. y?=w1862:bool)
        n1235 = And(x="Trap 1 ON", y=w1867) -> (x .and. y?=w1865:bool)
        n1236 = Multiply(x=w1879, y=w1890) -> (x*y=w1887:dbl)
        n1237 = Multiply(x=w1889, y=w1878) -> (x*y=w1885:dbl)
        n1238 = Multiply(x=w1888, y=w1877) -> (x*y=w1886:dbl)
        n1239 = Multiply(x=w1891, y=w1876) -> (x*y=w1894:dbl)
        n1240 = Multiply(x=w1892, y=w1875) -> (x*y=w1895:dbl)
        n1241 = Multiply(x=w1893, y=w1874) -> (x*y=w1896:dbl)
        n1242 = call "set RF board amplitude - interlace.vi"("Board 2 Amplitude Limits"=w1860, "Board 1 Amplitude Limits"=w1861, "FPGA VI Reference In"=w1859, "Board 2 Amplitude 3 (%)"=w1896, "Board 1 Amplitude 3 (%)"=w1886, "Board 2 Amplitude 2 (%)"=w1895, "Board 2 Amplitude 1 (%)"=w1894, "Board 1 Amplitude 2 (%)"=w1885, "Board 1 Amplitude 1 (%)"=w1887) -> ("error out"=w1869:errorcluster, "FPGA VI Reference Out"=w1870:T31)  [unwired: 1 in]
        n1243 = xnode "Read/Write Control"("FPGA VI Reference In"=w1870, "error in"=w1869, "FB On/Off Set 1"=w1865, "FB On/Off Set 2"=w1862) -> ("error out"=w1868:errorcluster)  [unwired: 1 out]
      }
      event "Load parameters": Value Change {
        n1244 = event-data() -> ()  [unwired: 7 out]
        n1245 = property on="Saved AOD Raster Scan Parameter Sets" class="Arr (strict)"() -> ("Index Values"=w1907:u32[])  [unwired: 2 in, 2 out]
        n1246 = Index Array(array=w1907, index=0) -> (element=w1904:u32)
        n1247 = local write "Load parameters"(FALSE ("Load parameters")) -> ()
        n1248 = Index Array(array="Saved AOD Raster Scan Parameter Sets", index=w1904) -> (element=w1903:T42)
        n1249 = Unbundle By Name(w1903) -> ("Scan Range AOD (nm) 2"=w1902:dbl, "Step Size AOD (nm) 2"=w1901:dbl, "Scan Speed AOD (nm/s) 2"=w1900:dbl, "Number of scans (AOD) 2"=w1899:u16)
        n1250 = flat-sequence {
          tunnel: w1902 -> [w1910]
          tunnel: w1901 -> [w1909]
          tunnel: w1900 -> [w1908]
          tunnel: w1899 -> [w1911]
          frame #0 {
            n1251 = local write "Scan Speed (nm/s)"(w1908) -> ()
            n1252 = local write "Scan Range (nm)"(w1910) -> ()
            n1253 = local write "Step Size (nm)"(w1909) -> ()
          }
          frame #1 {
            n1254 = property on="Number of F/B Scans (AOD)" class="DigNum (strict)"("Val(Sgnl)"=w1911) -> ()  [unwired: 2 in, 2 out]
          }
        }
      }
      event "Trap 1 (ON/OFF)", "Trap 2 (ON/OFF)": Value Change {
        n1255 = event-data() -> ()  [unwired: 7 out]
        n1256 = flat-sequence {
          tunnel: [w1921] -> w1916
          tunnel: w1916 -> [w1936]
          tunnel: [w1922] -> w1912
          frame #0 {
            n1257 = local read "Trap 1 ON"() -> (w1921:bool)
          }
          frame #1 {
            n1258 = Exclusive Or(1:w1936, 2:"Trap 1 (ON/OFF)") -> (0:w1929:bool)
            n1259 = Select(t="on", s="Trap 2 (ON/OFF)", f="off") -> (s? t:f=w1928:string)
            n1260 = Select(t="on", s="Trap 1 (ON/OFF)", f="off") -> (s? t:f=w1924:string)
            n1261 = Build Array("trap 1 ", w1924) -> (w1923:string[])
            n1262 = Build Array("trap 2 " ("f"), w1928) -> (w1926:string[])
            n1263 = Select(t=w1923, s=w1929, f=w1926) -> (s? t:f=w1922:string[])
            n1264 = property on="Trap 1 ON" class="Bool (strict)"("Val(Sgnl)"="Trap 1 (ON/OFF)") -> ()  [unwired: 2 in, 2 out]
            n1265 = property on="Trap 2 ON" class="Bool (strict)"("Val(Sgnl)"="Trap 2 (ON/OFF)") -> ()  [unwired: 2 in, 2 out]
          }
        }
        n1266 = local read "Saving..."() -> (w1915:bool)
        n1267 = local read "Save Event Log?"() -> (w1914:bool)
        n1268 = And(x=w1915, y=w1914) -> (x .and. y?=w1913:bool)
        n1269 = case shown="True" w1913 {
          tunnel: w1912 -> [_ w1920]
          frame False {
          }
          frame True {
            n1270 = local read "Time (s)"() -> (w1917:dbl)
            n1271 = local read "log file ref"() -> (w1919:refnum<file>)
            n1272 = Concatenate Strings(w1920) -> (w1918:string)
            n1273 = call "write to event log.vi"("log file ref"=w1919, "time"=w1917, "input string"=w1918) -> ()  [unwired: 8 in]
          }
        }
      }
      event "DIO count 1 (ticks)", "DIO count 2 (ticks)", "DIO count 3 (ticks)", "Interlace", "Number Interlace Sets", "Not-Interlacing Set", "BD 1 Delay (ticks)", "BD 2 Delay (Ticks)", "Next trap write delay (ticks)", "XY phase ext loop method", "Amp switch delay 2", "BD 2 Delay (Ticks) 2", "BD 1 Delay (ticks) 2": Value Change {
        n1274 = event-data() -> ()  [unwired: 7 out]
        n1275 = local read "DIO count 3 (ticks)"() -> (w1951:u16)
        n1276 = local read "DIO count 1 (ticks)"() -> (w1953:u16)
        n1277 = local read "DIO count 2 (ticks)"() -> (w1952:u16)
        n1278 = To Unsigned Byte Integer(number="Not-Interlacing Set") -> (unsigned 8bit integer=w1942:u8)
        n1279 = Add(x=w1942, y=u8 1) -> (x+y=w1946:u8)
        n1280 = xnode "Read/Write Control"("FPGA VI Reference In"=w1937, "DIO count 1 (ticks)"=w1953, "DIO count 2 (ticks)"=w1952, "DIO count 3 (ticks)"=w1951, "Interlace ON/OFF"="Interlace", "Number Interlace Cycles"="Number Interlace Sets", "Interlace Off Parameters"=w1946, "BD 1 Delay (ticks)"="BD 1 Delay (ticks)", "BD 2 Delay (Ticks)"="BD 2 Delay (Ticks)", "Next trap write delay (ticks)"="Next trap write delay (ticks)") -> ("error out"=w1955:errorcluster)  [unwired: 1 in, 1 out]
        n1281 = Build Array(w1953, w1952, w1951) -> (w1944:u16[])
        n1282 = Split 1D Array(array=w1944, index="Number Interlace Sets") -> (first subarray=w1954:u16[])  [unwired: 1 out]
        n1283 = Index Array(array=w1944, index=w1942) -> (element=w1943:u16)
        n1284 = Add Array Elements(numeric array=w1954) -> (sum=w1948:u16)
        n1285 = Select(t=w1948, s="Interlace", f=w1943) -> (s? t:f=→"Total Counts (ticks)":u16)
      }
      event "Reset Feedback": Value Change {
        n1286 = event-data() -> ()  [unwired: 7 out]
        n1287 = Unbundle By Name("Reset Feedback") -> ("Set 1"=w1959:bool, "Set 2"=w1958:bool)
        n1288 = xnode "Read/Write Control"("FPGA VI Reference In"=w1956, "FB Reset Set 1"=w1959, "FB Reset Set 2"=w1958) -> ("error out"=w1957:errorcluster)  [unwired: 1 in, 1 out]
      }
      event "Trap intensity output range", "Trap Intensity PID Gains": Value Change {
        n1289 = event-data() -> ()  [unwired: 7 out]
        n1290 = xnode "Read/Write Control"("FPGA VI Reference In"=w1963, "FB Gains"="Trap Intensity PID Gains", "FB output range"="Trap intensity output range") -> ("error out"=w1964:errorcluster)  [unwired: 1 in, 1 out]
      }
      event "AI2 to Setpoint", "Setpoints (V)": Value Change {
        n1291 = event-data() -> ()  [unwired: 7 out]
        n1292 = xnode "Read/Write Control"("FPGA VI Reference In"=w1965) -> ("FPGA VI Reference Out"=w1968:T31, "error out"=w1967:errorcluster, "AI2 Y Sum Set 1"=w1975:i16, "AI2 Y Sum Set 2"=w1974:i16)  [unwired: 1 in]
        n1293 = Cluster To Array(cluster="AI2 to Setpoint") -> (array=w1978:bool[])
        n1294 = local read "AI2 (V)"() -> (w1976:cluster{"Set 1":dbl, "Set 2":dbl})
        n1295 = Or Array Elements(Boolean array=w1978) -> (logical OR=w1979:bool)
        n1296 = Bundle By Name(cluster=w1976, "Set 1"=w1975, "Set 2"=w1974) -> (w1973:cluster{"Set 1":dbl, "Set 2":dbl})
        n1297 = Divide(x=w1973, y=3276.7) -> (x/y=w1972:cluster{"Set 1":dbl, "Set 2":dbl})
        "AI2 (V)" <- w1972
        n1298 = case shown="True" w1979 {
          tunnel: [w1982 w1999] -> w1971
          tunnel: "AI2 to Setpoint" -> [_ w1995]
          tunnel: "Setpoints (V)" -> [w1983 w1998]
          tunnel: w1972 -> [_ w1992]
          frame False {
            n1299 = Multiply(x=3276.7, y=w1983) -> (x*y=w1984:cluster{"Set 1":dbl, "Set 2":dbl})
